vi "remove tag by name.vi"(8 "error in":errorcluster, 10 "tag":string, 11 "tag collection in":refnum<class "tag collection.lvclass">) -> (0 "error out":errorcluster, 1 "removed tag":refnum<class "tag descriptor.lvclass">, 3 "tag collection out":refnum<class "tag collection.lvclass">)   [LabVIEW 2013, in "tag bus.lvlib" / "tag collection.lvclass"]
uses:
  tag collection.lvclass
  tag/tag descriptor.lvclass
  tag collection.lvclass/tag collection.ctl
  tag bus.lvlib
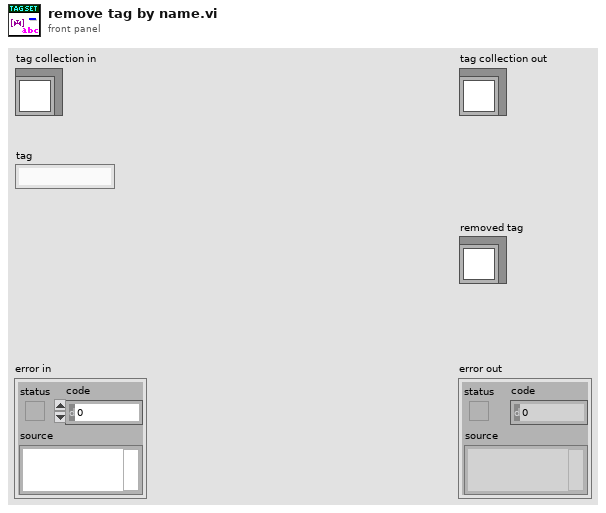
[diagram p1: front panel]
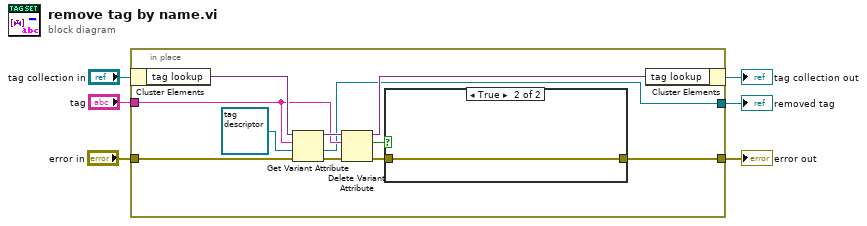
[diagram p0: block diagram]
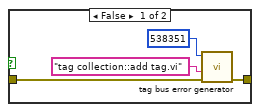
[diagram p2: hidden frame]
diagram:
  n1 = in-place {
    in-place-border: "error in" -> [w16]
    in-place-border: [w17] -> w3
    in-place-border: "tag" -> [w9]
    in-place-border: [w7] -> w1
    n2 = in-place-cluster #1("tag collection in") -> ("tag lookup"=w11:variant)
    n3 = Get Variant Attribute(Variant=w11, name=w9, default value (empty Variant)=refnum<class "tag descriptor.lvclass"> refnum ("tag"), error in=w16) -> (duplicate Variant=w10:variant, value=w7:refnum<class "tag descriptor.lvclass">, error out=w12:errorcluster)  [unwired: 1 out]
    n4 = Delete Variant Attribute(4:w12, 6:w9, 7:w10) -> (0:w15:errorcluster, 2:w14:bool, 3:w13:variant)
    n5 = case shown="True" w14 {
      tunnel: [w20 w22] -> w17
      tunnel: w15 -> [w21 w22]
      frame False {
        n6 = call "tag bus error generator.vi"("error in"=w21, "source"="tag collection::add tag.vi", "error code (0)"=538351) -> ("error out"=w20:errorcluster)  [unwired: 6 in]
      }
      frame True {
      }
    }
    n7 = in-place-cluster #1("tag lookup"=w13) -> (→"tag collection out":refnum<class "tag collection.lvclass">)
  }
  "error out" <- w3
  "removed tag" <- w1
